vi "CSM - Create CSM Palette at Root.vi"() -> ()   [LabVIEW 2017]
doc: "Create a CSM module palette at the root of the function palette."
uses:
  _Shared/CSM Shared.lvlib
panel:
  in  "Remove Button":bool
  in  "Add Button":bool
  out "String":string
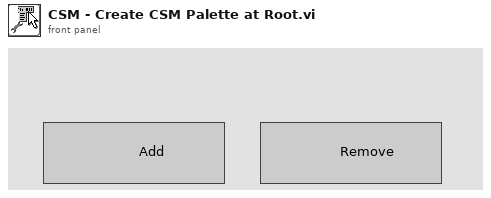
[diagram p1: front panel]
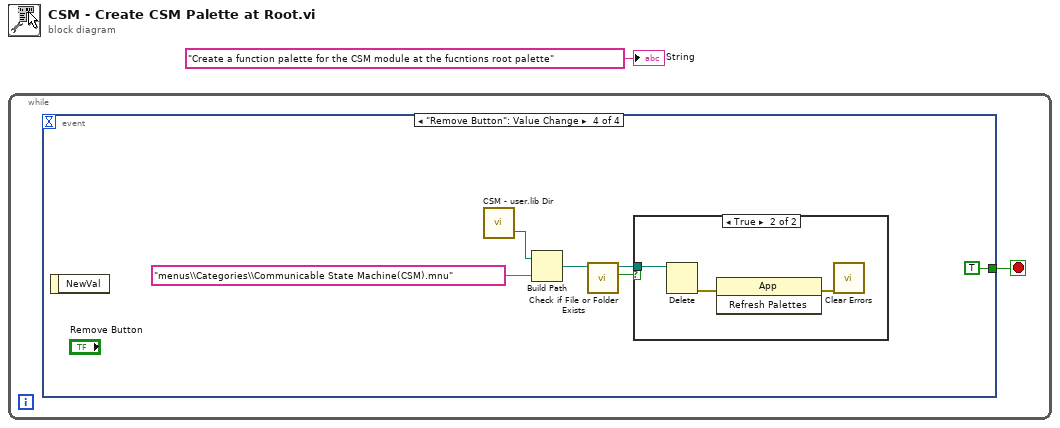
[diagram p0: block diagram]
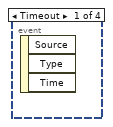
[diagram p2: hidden frame]
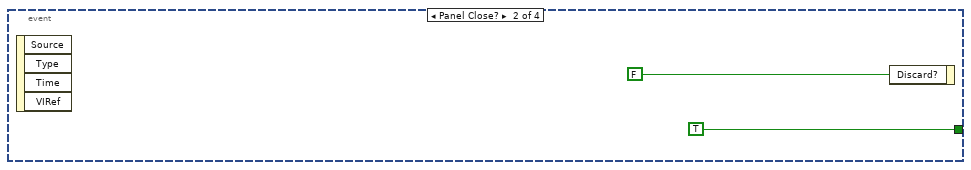
[diagram p3: hidden frame]
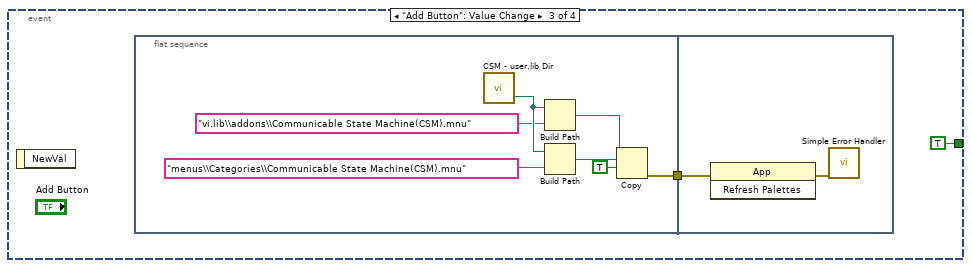
[diagram p4: hidden frame]
diagram:
  n1 = while {
    stop <- w2 stop-if-true
    n2 = event shown="[3] \"Remove Button\": Value Change" {
      selector: _ -> [_ _ _ _]
      dyn-events: _ -> [_ _ _ _]
      timeout: _ -> [_ _ _ _]
      tunnel: [_ TRUE ("Discard?") TRUE ("Discard?") TRUE ("Discard?")] -> w2
      event Timeout {
        n3 = event-data() -> ()  [unwired: 1 in, 3 out]
      }
      event Panel Close? {
        n4 = event-data() -> ()  [unwired: 1 in, 4 out]
        n5 = event-data("Discard?"=FALSE) -> ()  [unwired: 1 in, 1 out]
      }
      event "Add Button": Value Change {
        n6 = event-data() -> ()  [unwired: 1 in, 1 out]
        n7 = flat-sequence {
          tunnel: [w7] -> w6
          tunnel: w6 -> [w15]
          frame #0 {
            n8 = call "CSM - user.lib Dir.vi"() -> ("<LabVIEW>"=w13:path)  [unwired: 2 in, 1 out]
            n9 = Build Path(base path=w13, name or relative path="vi.lib\\addons\\Communicable State Machine(CSM).mnu") -> (appended path=w10:path)
            n10 = Build Path(base path=w13, name or relative path="menus\\Categories\\Communicable State Machine(CSM).mnu") -> (appended path=w9:path)
            n11 = Copy(9:TRUE ("overwrite (F)"), 10:w9, 11:w10) -> (0:w7:errorcluster)  [unwired: 2 in, 2 out]
          }
          frame #1 {
            n12 = invoke class="App" method="Refresh Palettes"(error in=w15) -> (error out=w14:errorcluster)  [unwired: 2 in, 2 out]
            n13 = call <vilib>:"Simple Error Handler.vi"("error in (no error)"=w14) -> ()  [unwired: 4 in, 5 out]
          }
        }
      }
      event "Remove Button": Value Change {
        n14 = event-data() -> ()  [unwired: 1 in, 1 out]
        n15 = call "CSM - user.lib Dir.vi"() -> ("<LabVIEW>"=w20:path)  [unwired: 2 in, 1 out]
        n16 = Build Path(base path=w20, name or relative path="menus\\Categories\\Communicable State Machine(CSM).mnu") -> (appended path=w17:path)
        n17 = call <vilib>:"Check if File or Folder Exists.vi"("path"=w17) -> ("file or folder exists?"=w19:bool, "dup path"=w18:path)  [unwired: 8 in, 1 out]
        n18 = case shown="True" w19 {
          tunnel: w18 -> [_ w23]
          frame False {
          }
          frame True {
            n19 = Delete(path (use dialog)=w23) -> (error out=w24:errorcluster)  [unwired: 4 in, 2 out]
            n20 = invoke class="App" method="Refresh Palettes"(error in=w24) -> (error out=w22:errorcluster)  [unwired: 2 in, 2 out]
            n21 = call <vilib>:"Clear Errors.vi"("error in (no error)"=w22) -> ()  [unwired: 5 in, 2 out]
          }
        }
      }
    }
  }
  "String" <- "Create a function palette for the CSM module at the fucntions root palette" ("String")
